vi "TSM SSC Digital PPMU Source Voltage Per-Site Per-Pin.vi"(0 "Digital TSM In":T1, 5 "Per-Site Per-Pin Source Voltages (V)":dbl[][](array[numeric]) format="%#_6p", 7 "Current Limit Range (A)":dbl format="%#_6p", 11 "error in":errorcluster) -> (4 "Digital TSM Out":T1, 15 "error out":errorcluster)   [LabVIEW 2019]
doc: "Sources per-site per-pin voltages from the PPMU to the specified pins connected to each site. This function takes in an array of voltages where rows correspond to sites and columns correspond to pins."
uses:
  TSM/TSM SSC Digital.ctl
  <vilib>/NI_TestStand_SemiconductorModule/NI_TestStand_Semiconductor_Module.lvlibp/PinMap/Digital Pattern/PinQueryContext/DigitalPatternPinQueryContext.lvclass
  SSC Digital/SSC Digital.ctl
  <instrlib>/niDigital/niDigital.llb/niDigital Output Function.ctl
  1a9f9ff5-721a-42b6-b454-8659b893b2e8.vi
  Shared SubVIs/Trim Whitespace [Inlined].vi
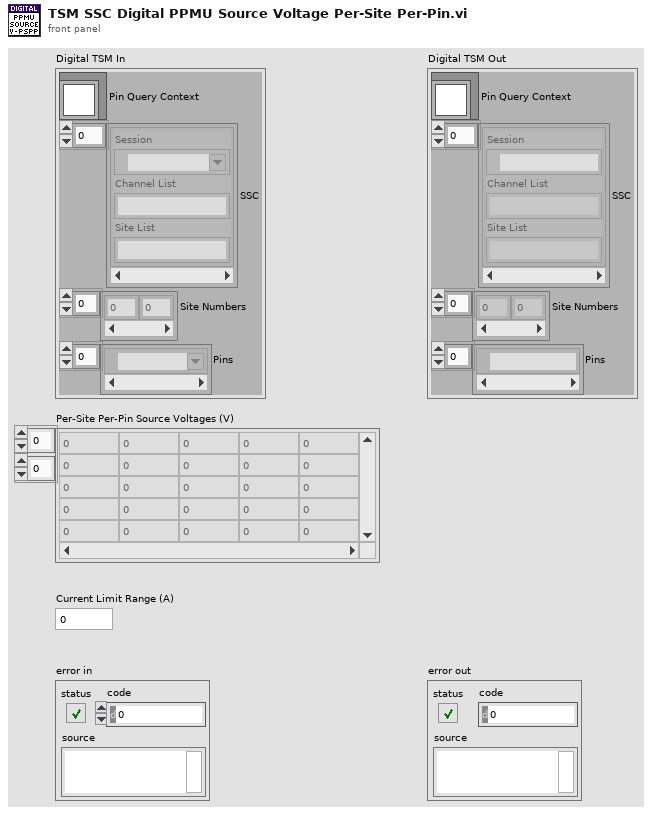
[diagram p1: front panel]
types:
  T1 = typedef "TSM SSC Digital.ctl" = cluster{"Pin Query Context":refnum<class "DigitalPatternPinQueryContext.lvclass">, "SSC":T2[], "Site Numbers":i32[], "Pins":tag[]}
  T2 = typedef "SSC Digital.ctl" = cluster{"Session":refnum<k15>, "Channel List":string, "Site List":string}
  T3 = typedef "Digital 2D Location.ctl" = cluster{"Row":i32, "Col":i32}
  T4 = typedef "niDigital Output Function.ctl" = i32
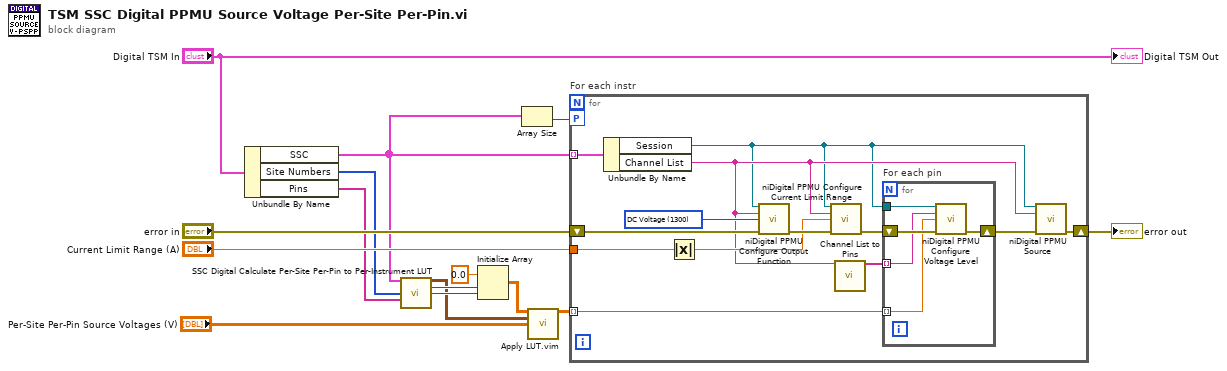
[diagram p0: block diagram]
diagram:
  n1 = Unbundle By Name("Digital TSM In") -> ("SSC"=w1:T2[], "Site Numbers"=w7:i32[], "Pins"=w6:tag[])
  n2 = call "SSC Digital Calculate Per-Site Per-Pin to Per-Instrument LUT.vi"("Digital SSC In"=w1, "Sites"=w7, "Pins"=w6) -> ("Per-Site Per-Pin to Per-Instrument LUT"=w10:T3[][], "Instrument Count"=w13:i32, "Max Sites on Instrument"=w12:i32)  [unwired: 10 in]
  n3 = Initialize Array(0.0 ("element"), w13, w12) -> (w11:dbl[][])
  n4 = Array Size(array=w1) -> (size(s)=w2:i32)
  n5 = call "Apply LUT.vim"("Initialized Array"=w11, "LUT"=w10, "Results to Apply LUT to"="Per-Site Per-Pin Source Voltages (V)") -> ("Array Out"=w9:dbl[][])  [unwired: 12 in]
  n6 = for "For each instr" {
    tunnel: "Current Limit Range (A)" -> [w27]
    workers-P: w2 -> [_]
    tunnel: w1 -> [w18] mode=indexing
    tunnel: w9 -> [w20] mode=indexing
    shift-right: [w26] -> w3
    shift-left: "error in" -> [w28]
    w23 = T4 1300 items=["DC Voltage"=1300, "DC Current"=1301] ("output function")
    n7 = Unbundle By Name(w18) -> ("Session"=w16:refnum<k15>, "Channel List"=w17:string)
    n8 = Absolute Value(x=w27) -> (abs(x)=w22:dbl)
    n9 = call <instrlib>:"niDigital PPMU Configure Output Function.vi"("instrument handle"=w16, "channel list"=w17, "output function"=w23, "error in"=w28) -> ("error out"=w25:errorcluster)  [unwired: 10 in, 1 out]
    n10 = call <instrlib>:"niDigital PPMU Configure Current Limit Range.vi"("instrument handle"=w16, "channel list"=w17, "current limit range (A)"=w22, "error in"=w25) -> ("error out"=w24:errorcluster)  [unwired: 10 in, 1 out]
    n11 = call "Channel List to Pins.vi"("Channel List"=w17) -> ("Sites and Pins"=w19:string[])  [unwired: 12 in, 2 out]
    n12 = for "For each pin" {
      shift-right: [w31] -> w21
      shift-left: w24 -> [w33]
      tunnel: w19 -> [w30] mode=indexing
      tunnel: w20 -> [w29] mode=indexing
      tunnel: w16 -> [w32]
      n13 = call <instrlib>:"niDigital PPMU Configure Voltage Level.vi"("instrument handle"=w32, "channel list"=w30, "voltage level (V)"=w29, "error in"=w33) -> ("error out"=w31:errorcluster)  [unwired: 10 in, 1 out]
    }
    n14 = call <instrlib>:"niDigital PPMU Source.vi"("instrument handle"=w16, "channel list"=w17, "error in"=w21) -> ("error out"=w26:errorcluster)  [unwired: 11 in, 1 out]
  }
  "error out" <- w3
  "Digital TSM Out" <- "Digital TSM In"
